vi "MP-285_data_decode.vi"(8 "error in (no error)":errorcluster, 9 "length":i32 min=0, 10 "offset":i32 min=0, 11 "encoded data string in":string) -> (0 "error out":errorcluster, 1 "decoded data":i32, 3 "encoded data string out":string)   [LabVIEW 2010, in "StageMG100204SutterMP285.lvclass"]
uses:
  StageMG100204SutterMP285.lvclass
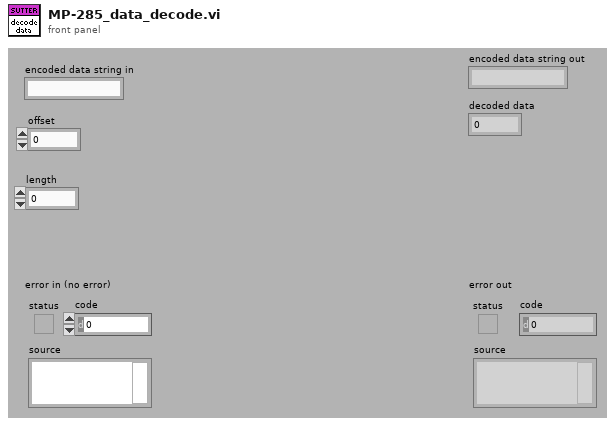
[diagram p1: front panel]
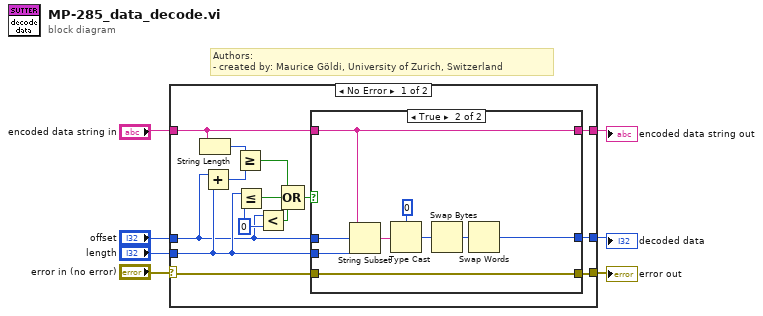
[diagram p0: block diagram]
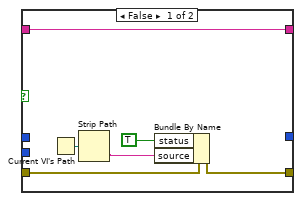
[diagram p2: hidden frame]
diagram:
  # "Authors: \n- created by: Maurice Göldi, University of Zurich, Switzerland"
  n1 = case shown="No Error" "error in (no error)" {
    selector: "error in (no error)" -> [w15 w38]
    tunnel: [w14 w38] -> w6
    tunnel: [w13 w37] -> w5
    tunnel: "encoded data string in" -> [w8 w37]
    tunnel: [w12 _] -> w3
    tunnel: "offset" -> [w10 _]
    tunnel: "length" -> [w11 _]
    frame No Error {
      w18 = 0 ("offset")
      n2 = String Length(string=w8) -> (length=w16:i32)
      n3 = Add(x=w10, y=w11) -> (x+y=w17:i32)
      n4 = Greater Or Equal?(x=w16, y=w17) -> (x >= y?=w21:bool)
      n5 = Less Or Equal?(x=w11, y=w18) -> (x <= y?=w20:bool)
      n6 = Less?(x=w10, y=w18) -> (x < y?=w19:bool)
      n7 = Compound Arithmetic op=OR(w21, w20, w19) -> (w9:bool)
      n8 = case shown="True" w9 {
        tunnel: w15 -> [w26 w32]
        tunnel: [w25 w32] -> w14
        tunnel: w8 -> [w27 w28]
        tunnel: w10 -> [_ w31]
        tunnel: w11 -> [_ w30]
        tunnel: [_ w29] -> w12
        tunnel: [w27 w28] -> w13
        frame False {
          n9 = Current VI's Path() -> (path=w23:path)
          n10 = Strip Path(path=w23) -> (name=w22:string)  [unwired: 1 out]
          n11 = Bundle By Name(cluster=w26, "status"=TRUE, "source"=w22) -> (w25:errorcluster)
        }
        frame True {
          n12 = String Subset(string=w28, offset (0)=w31, length (rest)=w30) -> (substring=w34:string)
          n13 = Type Cast(type=0, x=w34) -> (*(type *) &x=w35:i32)
          n14 = Swap Bytes(anything=w35) -> (byte swapped=w36:i32)
          n15 = Swap Words(1:w36) -> (0:w29:i32)
        }
      }
    }
    frame Error {
    }
  }
  "error out" <- w6
  "encoded data string out" <- w5
  "decoded data" <- w3
